vi "PL_Spectrum_detailed.vi"() -> ()   [LabVIEW 2012]
uses:
  <vilib>/Utility/file.llb/Write To Spreadsheet File (DBL).vi
  <vilib>/Instr/_visa.llb/VISA Configure Serial Port (Instr).vi
  <vilib>/Analysis/baseanly.llb/Mean (DBL).vi
  <vilib>/Analysis/NI_AALBase.lvlib
panel:
  out "Filter Position":string
  out "Current Wavelength (nm)":string
  out "XY Graph":cluster{"Y":dbl[], "Y":dbl[]}[](graph)
  in  "End Wavelength (nm)":dbl
  in  "Start Wavelength (nm)":dbl
  in  "Resolution (nm)":dbl
  in  "Detector Input":T1
  in  "stop (T)":bool=TRUE
  in  "Resource name":refnum<visa-resource-name>
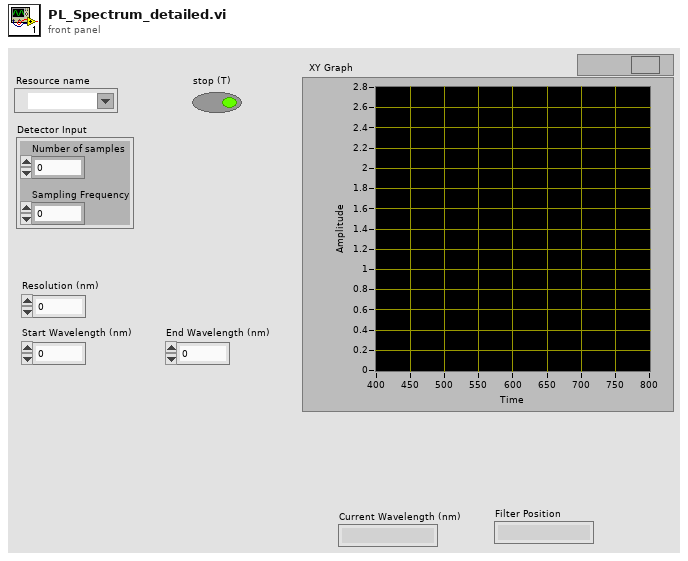
[diagram p1: front panel]
types:
  T1 = cluster{"Number of samples":i32, "Sampling Frequency":dbl}
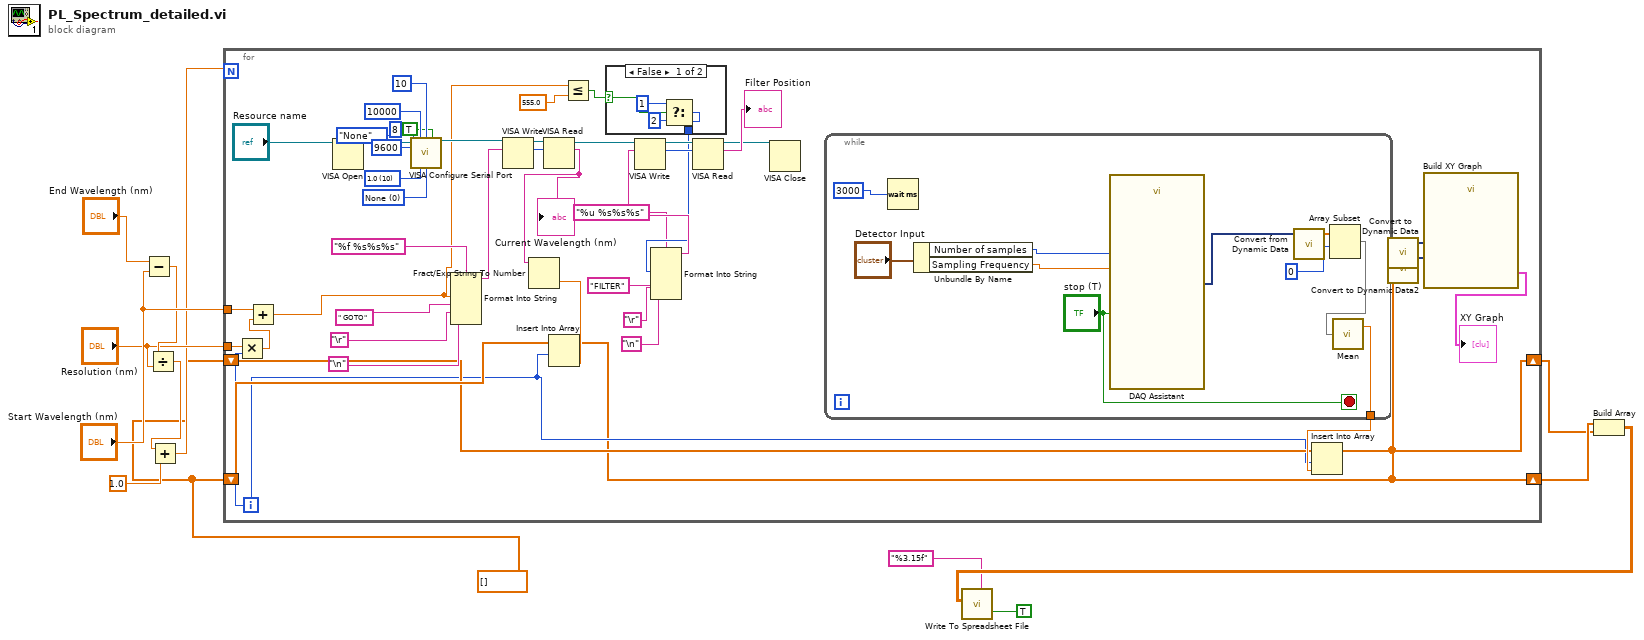
[diagram p0: block diagram]
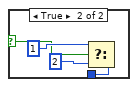
[diagram p2: hidden frame]
diagram:
  w5 = dbl[] [] ("array")
  n1 = Subtract(x="End Wavelength (nm)", y="Start Wavelength (nm)") -> (x-y=w10:dbl)
  n2 = Divide(x=w10, y="Resolution (nm)") -> (x/y=w8:dbl)
  n3 = Add(x=w8, y=1.0) -> (x+y=w6:dbl)
  n4 = for {
    N: w6 -> [_]
    shift-right: [w32] -> w4
    shift-left: w5 -> [w40]
    tunnel: "Resolution (nm)" -> [w39]
    tunnel: "Start Wavelength (nm)" -> [w38]
    shift-right: [w30] -> w3
    shift-left: w5 -> [w35]
    i -> [w34]
    w48 = u16 0 items=["None", "XON/XOFF", "RTS/CTS", "XON/XOFF & RTS/CTS", "DTR/DSR", "XON/XOFF & DTR/DSR"] ("flow control (0:none)")
    w49 = u16 10 items=["1.0"=10, "1.5"=15, "2.0"=20] ("stop bits (10: 1 bit)")
    n5 = Multiply(x=w39, y=w34) -> (x*y=w41:dbl)
    n6 = Add(x=w38, y=w41) -> (x+y=w28:dbl)
    n7 = VISA Open(VISA resource name="Resource name") -> (VISA resource name=w53:refnum<visa-resource-name>)  [unwired: 4 in, 1 out]
    n8 = call-poly "VISA Configure Serial Port"("VISA resource name"=w53, "timeout (10sec)"=u32 10000, "termination char\n(0xA = '\\n' = LF)"=u8 10 ("termination char\n(0xA = '\\n' = LF)"), "Enable Termination\nChar (T)"=TRUE ("Enable Termination\nChar (T)"), "baud rate (9600)"=u32 9600, "data bits (8)"=u16 8, "parity (0:none)"=enum16{"None", "Odd", "Even", "Mark", "Space"}."None", "stop bits (10: 1 bit)"=w49, "flow control (0:none)"=w48) -> ("VISA resource name out"=w43:refnum<visa-resource-name>)  [unwired: 5 in, 1 out]
    n9 = Format Into String(format string="%f %s%s%s", w28, " GOTO" ("String"), "\r", "\n") -> (resulting string=w44:string)  [unwired: 2 in, 1 out]
    n10 = VISA Write(VISA resource name=w43, write buffer=w44) -> (VISA resource name out=w55:refnum<visa-resource-name>, return count=w54:u32)  [unwired: 1 in, 1 out]
    n11 = VISA Read(VISA resource name=w55, byte count=w54) -> (VISA resource name out=w22:refnum<visa-resource-name>, read buffer=w26:string)  [unwired: 1 in, 2 out]
    "Current Wavelength (nm)" <- w26
    n12 = Fract/Exp String To Number(string=w26) -> (number=w37:dbl)  [unwired: 3 in, 1 out]
    n13 = Insert Into Array(array=w40, index=w34, new element=w37) -> (w32:dbl[])
    n14 = Less Or Equal?(x=w28, y=555.0) -> (x <= y?=w24:bool)
    n15 = case shown="False" w24 {
      selector: w24 -> [w60 w65]
      tunnel: [w63 w64] -> w18
      frame False {
        n16 = Select(t=1, s=w60, f=2) -> (s? t:f=w63:i32)
      }
      frame True {
        n17 = Select(t=1, s=w65, f=2) -> (s? t:f=w64:i32)
      }
    }
    n18 = Format Into String(format string="%u %s%s%s", w18, "FILTER" ("input 2"), "\r", "\n") -> (resulting string=w23:string)  [unwired: 2 in, 1 out]
    n19 = VISA Write(VISA resource name=w22, write buffer=w23) -> (VISA resource name out=w20:refnum<visa-resource-name>, return count=w21:u32)  [unwired: 1 in, 1 out]
    n20 = VISA Read(VISA resource name=w20, byte count=w21) -> (VISA resource name out=w14:refnum<visa-resource-name>, read buffer=→"Filter Position":string)  [unwired: 1 in, 2 out]
    n21 = VISA Close(VISA resource name=w14) -> ()  [unwired: 1 in, 1 out]
    n22 = while {
      tunnel: [w73] -> w36
      stop <- "stop (T)" stop-if-true
      n23 = Wait (ms)(milliseconds to wait=u32 3000) -> ()  [unwired: 1 out]
      n24 = Unbundle By Name("Detector Input") -> ("Number of samples"=w70:i32, "Sampling Frequency"=w69:dbl)
      n25 = call "DAQ Assistant"("rate"=w69, "number of samples"=w70, "stop (T)"="stop (T)") -> ("data"=w77:dynamicdata)  [unwired: 14 in, 2 out]
      n26 = call "Convert from Dynamic Data"("Dynamic Data Type"=w77) -> ("Array"=w76:dbl[])  [unwired: 3 in]
      n27 = Array Subset(array=w76, index=0) -> (w75:dbl[])  [unwired: 1 in]
      n28 = call-poly <vilib>:"Mean.vi"("X"=w75) -> ("mean"=w73:dbl)  [unwired: 1 out]
    }
    n29 = Insert Into Array(array=w35, index=w34, new element=w36) -> (w30:dbl[])
    n30 = call "Convert to Dynamic Data"("Array"=w32) -> ("Dynamic Data Type"=w31:dynamicdata)  [unwired: 3 in]
    n31 = call "Convert to Dynamic Data2"("Array"=w30) -> ("Dynamic Data Type"=w29:dynamicdata)  [unwired: 3 in]
    n32 = call "Build XY Graph"("Y Input"=w29, "X Input"=w31) -> ("XY Graph"=→"XY Graph":cluster{"Y":dbl[], "Y":dbl[]}[])  [unwired: 8 in, 1 out]
  }
  n33 = Build Array(w4, w3) -> (w2:dbl[][])
  n34 = call-poly <vilib>:"Write To Spreadsheet File.vi"("transpose? (no:F)"=TRUE, "format (%.3f)"="%3.15f" ("format string"), "2D data"=w2) -> ()  [unwired: 5 in, 1 out]
